vi "CloseDevices_SE.vi"(8 "error in":errorcluster, 11 "Data Highway In":T1={"New Image"=refnum, "Session Out"="", "LIDAR VISA Name"="", "Phidget Device Out"=0, "Lidar Data"=[], "polar attributes"={"maximum"=0.0, "minimum"=0.0, "clip to min"=FALSE, "log?(F)"=FALSE, "grid color"=6710886, "plot color"=65280, "fmt and prec"={"format"=enum."Decimal", "precision"=0}, "visible section"=8}, "Debug Message"="", "Servo Angles"={"Angle X"=0.0, "Angle Y"=0.0}, "ColorPlane"=refnum, "Threshold"=refnum, "PartFilt"=refnum, "Processed Image"=refnum, "Magnitude"=[], "Direction"=[]} {"polar attributes"."minimum" format="%0.2f"; "polar attributes"."maximum" format="%0.2f"}) -> (0 "error out":errorcluster)   [LabVIEW 2014]
uses:
  controls/Data.ctl
  <vilib>/vision/Image Controls.llb/IMAQ Image.ctl
  <vilib>/userdefined/High Color/IMAQdx.ctl
  Program Files (x86)/National Instruments/LabVIEW 2014/instr.lib/Hokuyo URG Series/Hokuyo URG Series.lvlib
  <vilib>/vision/driver/NI_Vision_Acquisition_Software.lvlib
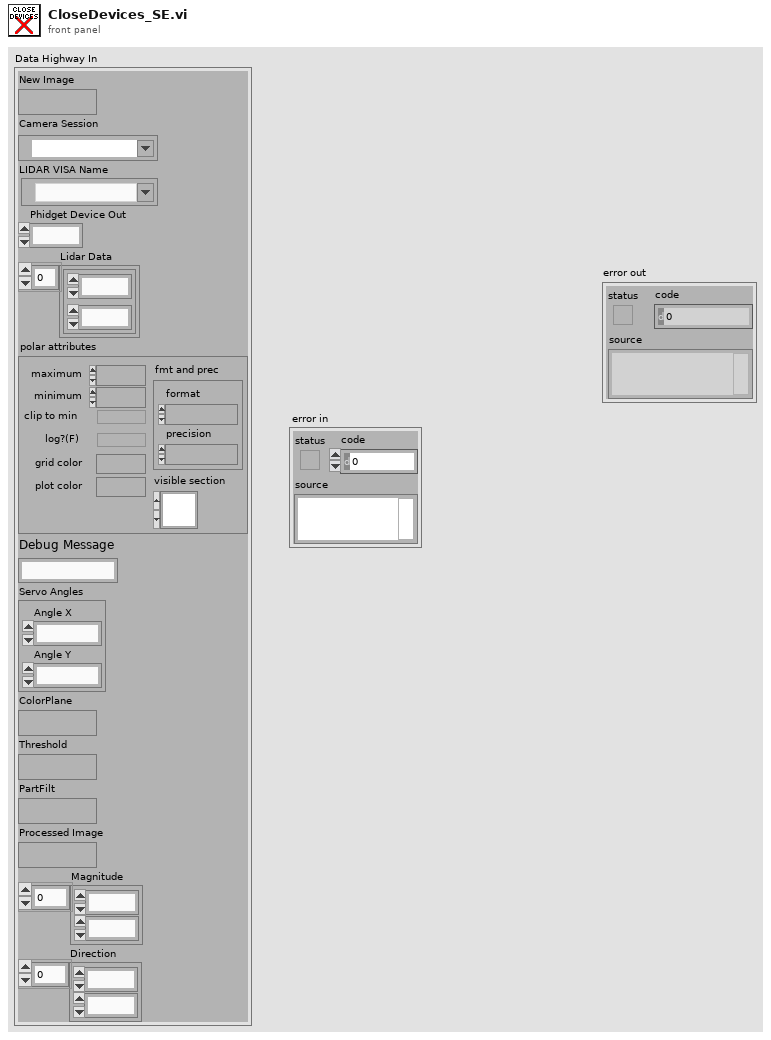
[diagram p1: front panel]
types:
  T1 = typedef "Data.ctl" = cluster{"New Image":T2, "Session Out":T3, "LIDAR VISA Name":refnum<visa-resource-name>, "Phidget Device Out":i32, "Lidar Data":cluster{dbl, dbl}[], "polar attributes":cluster{"maximum":dbl, "minimum":dbl, "clip to min":bool, "log?(F)":bool, "grid color":u32, "plot color":u32, "fmt and prec":cluster{"format":enum8{"Decimal", "Scientific", "Engineering", "Binary", "Octal", "Hex"}, "precision":u8}, "visible section":u16}, "Debug Message":string, "Servo Angles":cluster{"Angle X":dbl, "Angle Y":dbl}, "ColorPlane":T2, "Threshold":T2, "PartFilt":T2, "Processed Image":T2, "Magnitude":dbl[], "Direction":dbl[]}
  T2 = typedef "IMAQ Image.ctl" = refnum<image>
  T3 = typedef "IMAQdx.ctl" = refnum<k21>
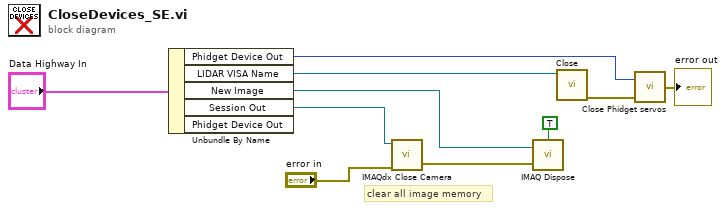
[diagram p0: block diagram]
diagram:
  # "clear all image memory"
  n1 = Unbundle By Name("Data Highway In") -> ("Phidget Device Out"=w1:i32, "LIDAR VISA Name"=w2:refnum<visa-resource-name>, "New Image"=w4:T2, "Session Out"=w3:T3)  [unwired: 1 out]
  n2 = call <vilib>:"IMAQdx Close Camera.vi"("error in"="error in", "Session In"=w3) -> ("error out"=w9:errorcluster)  [unwired: 9 out]
  n3 = call "IMAQ Dispose"("All Images? (No)"=TRUE, "Image"=w4, "error in (no error)"=w9) -> ()  [unwired: 4 out]
  n4 = call "Close.vi"("VISA resource name"=w2) -> ("error out"=w7:errorcluster)  [unwired: 10 in]
  n5 = call "Close Phidget servos.vi"("error in"=w7, "Device In"=w1) -> ("error out"=→"error out":errorcluster)
